vi "Compute FFT 64f.vi"(8 "Error In":errorcluster, 9 "Complex In":T5={"Device ID"=0, "Memeroy ID"=0, "Dimension"={"Depth"=0, "Height"=0, "Width"=0}, "Memory Type"=enum."64f"} {"Dimension"."Width" min=1; "Dimension"."Height" min=1; "Dimension"."Depth" min=1}, 10 "Real In":T5 {"Dimension"."Width" min=1; "Dimension"."Height" min=1; "Dimension"."Depth" min=1}, 11 "FFT Object":T1 {"Imag"."Dimension"."Width" min=1; "Imag"."Dimension"."Height" min=1; "Imag"."Dimension"."Depth" min=1; "Real"."Dimension"."Width" min=1; "Real"."Dimension"."Height" min=1; "Real"."Dimension"."Depth" min=1}) -> (0 "Error Out":errorcluster, 1 "Imag Out":T5 {"Dimension"."Width" min=1; "Dimension"."Height" min=1; "Dimension"."Depth" min=1}, 2 "Real Out":T5 {"Dimension"."Width" min=1; "Dimension"."Height" min=1; "Dimension"."Depth" min=1}, 3 "FFT Object Out":T1 {"Imag"."Dimension"."Width" min=1; "Imag"."Dimension"."Height" min=1; "Imag"."Dimension"."Depth" min=1; "Real"."Dimension"."Width" min=1; "Real"."Dimension"."Height" min=1; "Real"."Dimension"."Depth" min=1}, 4 "Time in ms":dbl)   [LabVIEW 2012, in "OpenCLV x64.lvlib"]
doc: "Computes the FFT based on the input plan provided. The Input Buffer <b>must</b> match those used to create the plan."
uses:
  OpenCLV x64.lvlib
  FFT Control.ctl
  Controls/Device ID.ctl
  FFT Types.ctl
  FFT Dimension.ctl
  Controls/Memory Object.ctl
  Controls/Memory ID.ctl
  User Controls/Array Dimensions.ctl
  Controls/Memory Type.ctl
  FFT Direction.ctl
  Error Checking/Add Error Functional Global.vi
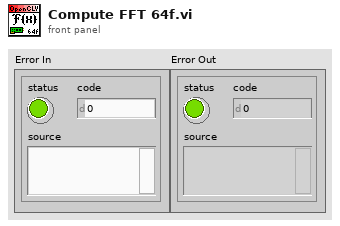
[diagram p1: front panel]
types:
  T1 = typedef "OpenCLV x64.lvlib/FFT Control.ctl" = cluster{"Device ID":T2, "FFT Types":T3, "FFT Dim":T4, "Real":T5, "Imag":T5, "FFT Plan":u64, "FFT Direction":T9}
  T2 = typedef "OpenCLV x64.lvlib/Device ID.ctl" = u64
  T3 = typedef "OpenCLV x64.lvlib/FFT Types.ctl" = enum16{"Real to Hermitian", "Hermitian to Real", "Complex to Complex"}
  T4 = typedef "OpenCLV x64.lvlib/FFT Dimension.ctl" = enum16{"1D FFT", "2D FFT", "3D FFT"}
  T5 = typedef "OpenCLV x64.lvlib/Memory Object.ctl" = cluster{"Device ID":T2, "Memeroy ID":T6, "Dimension":T7, "Memory Type":T8}
  T6 = typedef "OpenCLV x64.lvlib/Memory ID.ctl" = u64
  T7 = typedef "Array Dimensions.ctl" = cluster{"Depth":u64, "Height":u64, "Width":u64}
  T8 = typedef "OpenCLV x64.lvlib/Memory Type.ctl" = enum16{"32f", "u8", "i8", "u16", "i16", "u32", "i32", "64f"}
  T9 = typedef "OpenCLV x64.lvlib/FFT Direction.ctl" = enum16{"Forward", "Reverse"}
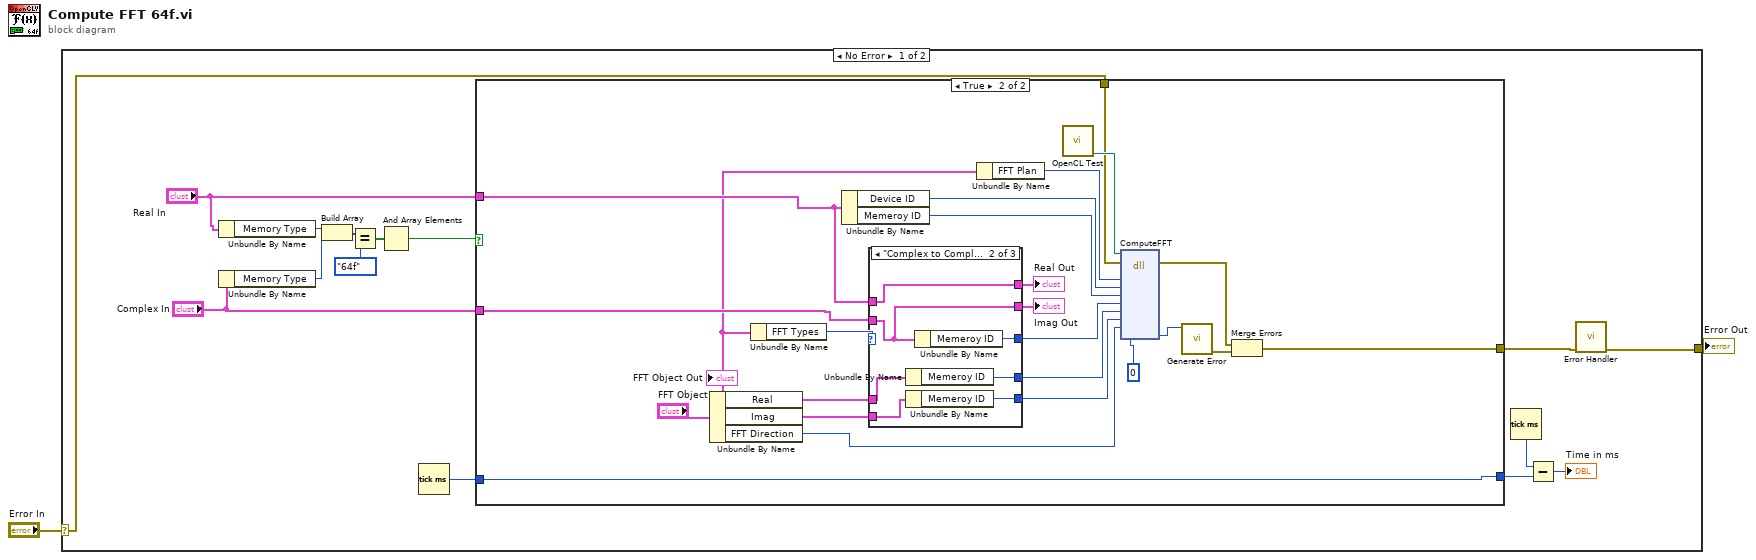
[diagram p0: block diagram]
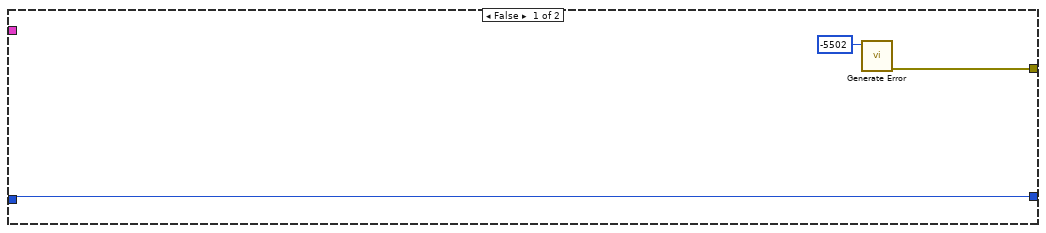
[diagram p2: hidden frame]
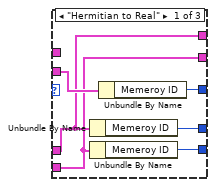
[diagram p3: hidden frame]
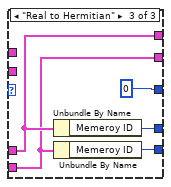
[diagram p4: hidden frame]
diagram:
  n1 = case shown="No Error" "Error In" {
    selector: "Error In" -> [w3 w62]
    tunnel: [w4 w62] -> w1
    frame No Error {
      n2 = Unbundle By Name("Real In") -> ("Memory Type"=w16:T8)
      n3 = Unbundle By Name("Complex In") -> ("Memory Type"=w17:T8)
      n4 = Build Array(w16, w17) -> (w15:T8[])
      n5 = Equal?(x=w15, y=Memory_Type."64f" ("Memory Type")) -> (x = y?=w13:bool[])
      n6 = And Array Elements(Boolean array=w13) -> (logical AND=w10:bool)
      n7 = Tick Count (ms)() -> (millisecond timer value=w7:u32)
      n8 = case shown="True" w10 {
        tunnel: [w20 w43] -> w5
        tunnel: "Real In" -> [_ w42]
        tunnel: "Complex In" -> [_ w41]
        tunnel: [w18 w22] -> w8
        tunnel: w7 -> [w18 w22]
        tunnel: w3 -> [_ w21]
        frame False {
          n9 = call "Generate Error.vi"("Error"=-5502) -> ("error out"=w20:errorcluster)  [unwired: 10 in]
        }
        frame True {
          n10 = Unbundle By Name("FFT Object") -> ("Real"=w30:T5, "Imag"=w29:T5, "FFT Direction"=w32:T9)
          n11 = Unbundle By Name("FFT Object") -> ("FFT Types"=w31:T3)
          n12 = Unbundle By Name(w42) -> ("Device ID"=w37:T2, "Memeroy ID"=w38:T6)
          n13 = case shown="\"Complex to Complex\"" w31 {
            tunnel: w30 -> [w45 w53 w58]
            tunnel: w29 -> [w44 w52 w57]
            tunnel: [w49 w56 w61] -> w26
            tunnel: [w48 w55 w60] -> w27
            tunnel: [w47 w54 T6 0 ("Memeroy ID")] -> w28
            tunnel: w41 -> [w46 w50 _]
            tunnel: w42 -> [_ w51 _]
            tunnel: [w45 w51 w58] -> w25
            tunnel: [w44 w50 w57] -> w24
            frame "Hermitian to Real" {
              n14 = Unbundle By Name(w45) -> ("Memeroy ID"=w48:T6)
              n15 = Unbundle By Name(w44) -> ("Memeroy ID"=w49:T6)
              n16 = Unbundle By Name(w46) -> ("Memeroy ID"=w47:T6)
            }
            frame "Complex to Complex" {
              n17 = Unbundle By Name(w53) -> ("Memeroy ID"=w55:T6)
              n18 = Unbundle By Name(w52) -> ("Memeroy ID"=w56:T6)
              n19 = Unbundle By Name(w50) -> ("Memeroy ID"=w54:T6)
            }
            frame "Real to Hermitian" {
              n20 = Unbundle By Name(w58) -> ("Memeroy ID"=w60:T6)
              n21 = Unbundle By Name(w57) -> ("Memeroy ID"=w61:T6)
            }
          }
          "Real Out" <- w25
          "Imag Out" <- w24
          n22 = Unbundle By Name("FFT Object") -> ("FFT Plan"=w36:u64)
          n23 = call "OpenCL Test.vi"() -> ("DLL To Use"=w23:path)  [unwired: 11 in]
          n24 = dll-call lib="C:/Users/bme-amcelroy-la/Desktop/OpenCLV/trunk/OpenCLV_x64_1.0/OpenCLV_x64.dll" fn="ComputeFFT"(path in=w23, error in=w21, "FFT Plan"=w36, "Labview Device"=w37, "Input Real"=w38, "Input Complex"=w28, "Output Real"=w27, "Output Complex"=w26, "Direction"=w32, "Error"=0) -> (error out=w34:errorcluster, "Error"=w40:i32)  [unwired: 9 in, 1 out]
          n25 = call "Generate Error.vi"("Error"=w40) -> ("error out"=w35:errorcluster)  [unwired: 10 in]
          n26 = Merge Errors(w34, w35) -> (w43:errorcluster)
          "FFT Object Out" <- "FFT Object"
        }
      }
      n27 = Tick Count (ms)() -> (millisecond timer value=w6:u32)
      n28 = Subtract(x=w6, y=w8) -> (x-y=→"Time in ms":u32)
      n29 = call-poly "Error Handler.vi"("Error In"=w5) -> ("Error Out"=w4:errorcluster)  [unwired: 10 in]
    }
    frame Error {
    }
  }
  "Error Out" <- w1
